vi "SSH Open.vi"(8 "Error In":errorcluster, 11 "Credentials":T1) -> (0 "Error Out":errorcluster, 2 "Connected?":bool, 3 "SSH Session":refnum<k24>)   [LabVIEW 2011, in "LMH-LINX.lvlib"]
uses:
  LMH-LINX.lvlib
  C:/Users/samkristoff/Desktop/Builds/2016_01_27/build/LabVIEW/vi.lib/MakerHub/LINX/Resources/Renci.SshNet.dll
  Resources/Renci.SshNet.dll
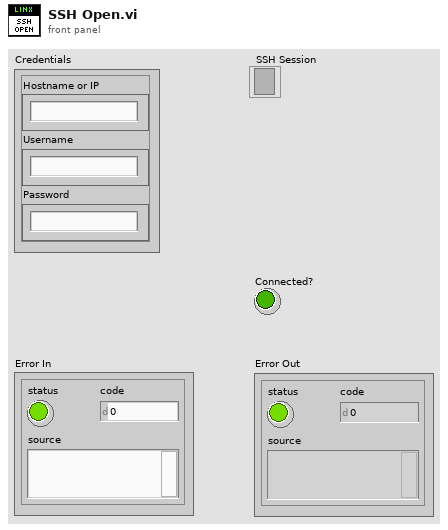
[diagram p1: front panel]
types:
  T1 = cluster{"Hostname or IP":string, "Username":string, "Password":string}
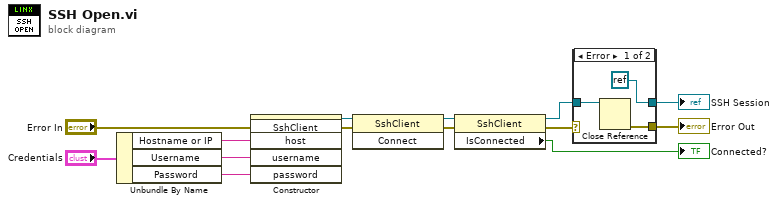
[diagram p0: block diagram]
diagram:
  n1 = Unbundle By Name("Credentials") -> ("Hostname or IP"=w7:string, "Username"=w6:string, "Password"=w5:string)
  n2 = constructor class="SshClient"(error in="Error In", "host"=w7, "username"=w6, "password"=w5) -> (reference out=w11:refnum<k24>, error out=w12:errorcluster)  [unwired: 2 in, 4 out]
  n3 = invoke class="SshClient" method="Connect"(reference=w11, error in=w12) -> (reference out=w14:refnum<k24>, error out=w13:errorcluster)  [unwired: 1 in, 1 out]
  n4 = property class="SshClient"(reference=w14, error in=w13) -> (reference out=w1:refnum<k24>, error out=w4:errorcluster, "IsConnected"=→"Connected?":bool)
  n5 = case shown="Error" w4 {
    selector: w4 -> [_ w18]
    tunnel: [w15 w18] -> w3
    tunnel: [refnum<k0> refnum w19] -> w2
    tunnel: w1 -> [w16 w19]
    frame Error {
      n6 = Close Reference(reference=w16) -> (error out=w15:errorcluster)  [unwired: 1 in]
    }
    frame No Error {
    }
  }
  "Error Out" <- w3
  "SSH Session" <- w2
